vi "Generate logfile path.vi"(8 "error in":errorcluster, 10 "Típus":string) -> (0 "error out":errorcluster, 2 "Log_Path":path)   [LabVIEW 2014]
panel:
  out "File name":string
  out "Folder exists?":bool
  out "Folder path":path
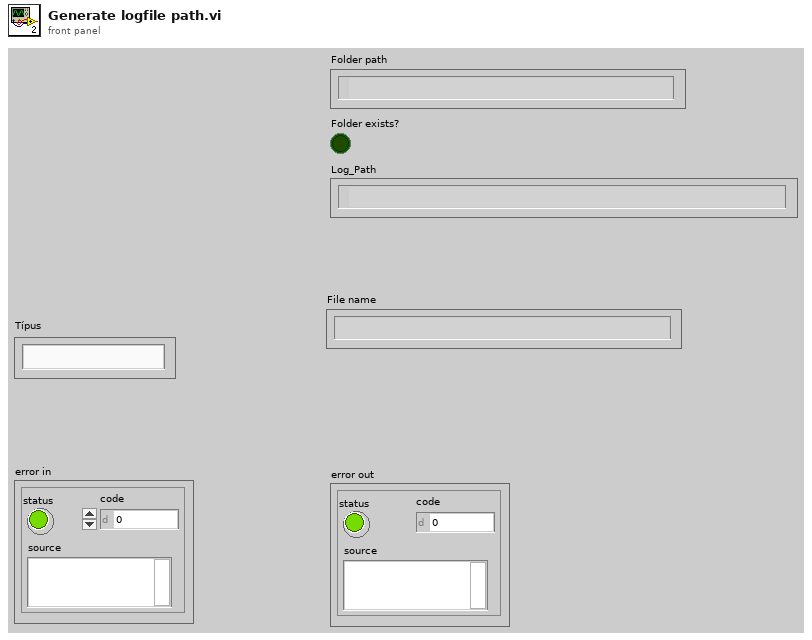
[diagram p1: front panel]
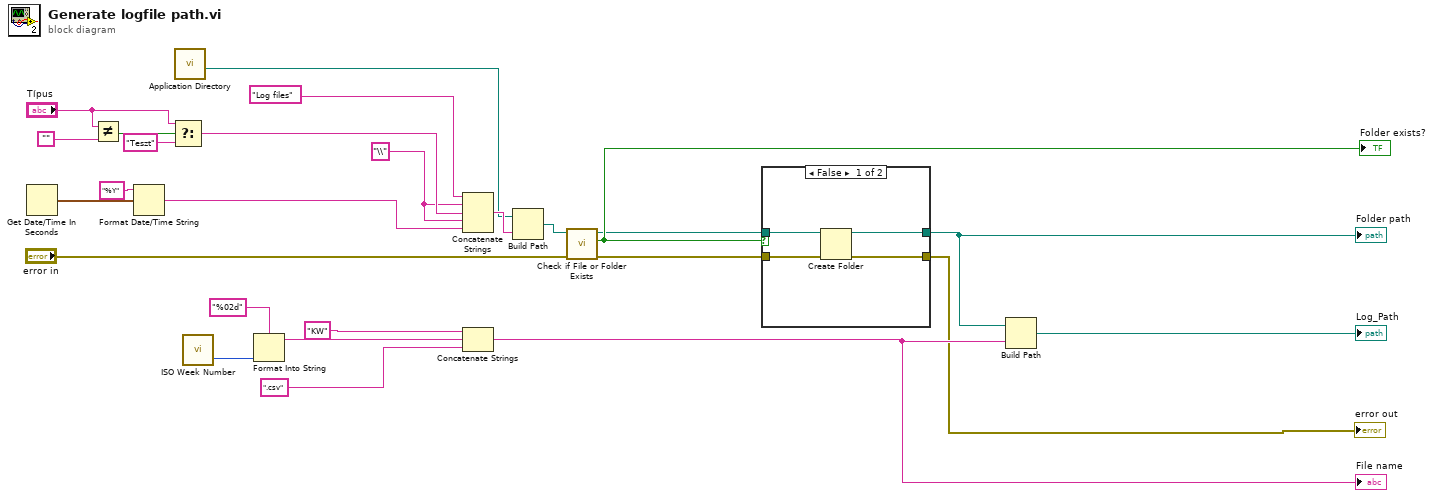
[diagram p0: block diagram]
diagram:
  w1 = "\\" ("prompt (Choose or enter file path)")
  n1 = Get Date/Time In Seconds() -> (seconds since 1Jan1904=w20:timestamp)
  n2 = Not Equal?(x="Típus", y="") -> (x != y?=w6:bool)
  n3 = Format Date/Time String(time format string (%c)="%Y", seconds (now)=w20) -> (date/time string=w12:string)  [unwired: 1 in]
  n4 = Select(t="Típus", s=w6, f="Teszt") -> (s? t:f=w3:string)
  n5 = call <vilib>:"Application Directory.vi"() -> ("Application Directory"=w11:path)
  n6 = call "ISO Week Number.vi"() -> ("ISO week"=w14:i32)  [unwired: 2 out]
  n7 = Format Into String(format string="%02d", w14) -> (resulting string=w9:string)  [unwired: 2 in, 1 out]
  n8 = Concatenate Strings("Log files" ("prompt (Choose or enter file path)"), w1, w3, w1, w12) -> (w18:string)
  n9 = Concatenate Strings("KW" ("string"), w9, ".csv" ("string")) -> (w22:string)
  "File name" <- w22
  n10 = Build Path(base path=w11, name or relative path=w18) -> (appended path=w17:path)
  n11 = call <vilib>:"Check if File or Folder Exists.vi"("error in (no error)"="error in", "path"=w17) -> ("error out"=w15:errorcluster, "file or folder exists?"=w25:bool, "dup path"=w16:path)  [unwired: 7 in]
  "Folder exists?" <- w25
  n12 = case shown="False" w25 {
    tunnel: w16 -> [w30 w32]
    tunnel: [w27 w32] -> w24
    tunnel: w15 -> [w29 w31]
    tunnel: [w28 w31] -> w21
    frame False {
      n13 = Create Folder(path (use dialog)=w30, error in=w29) -> (created path=w27:path, error out=w28:errorcluster)  [unwired: 1 in, 1 out]
    }
    frame True {
    }
  }
  "Folder path" <- w24
  "error out" <- w21
  n14 = Build Path(base path=w24, name or relative path=w22) -> (appended path=→"Log_Path":path)
